vi "Focus Gray Image Stack.vi"(4 "Height Map":T1, 6 "Focused Image":T1, 8 "error in (no error)":errorcluster, 10 "Kernel Size":i32, 11 "Image Stack":T1[](array[typedef])) -> (0 "error out":errorcluster, 2 "Height Map":T1(plugin-control), 3 "Focused Image":T1(plugin-control))   [LabVIEW 2013]
uses:
  <vilib>/vision/Image Controls.llb/IMAQ Image.ctl
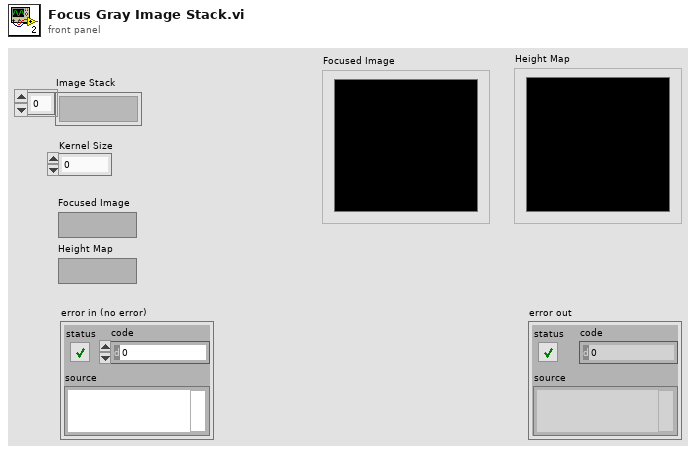
[diagram p1: front panel]
types:
  T1 = typedef "IMAQ Image.ctl" = refnum<image>
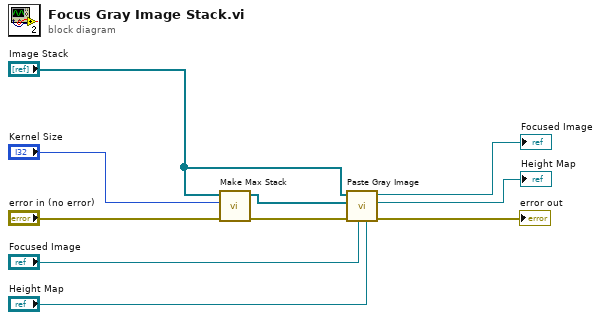
[diagram p0: block diagram]
diagram:
  n1 = call "Make Max Stack.vi"("error in (no error)"="error in (no error)", "Kernel Size"="Kernel Size", "Image Stack"="Image Stack") -> ("error out"=w10:errorcluster, "Max Stack"=w9:T1[])  [unwired: 7 in]
  n2 = call "Paste Gray Image.vi"("Height Map"="Height Map", "Focused Image"="Focused Image", "error in (no error)"=w10, "Max Image Stack"=w9, "Image Stack"="Image Stack") -> ("error out"=→"error out":errorcluster, "Height Map"=→"Height Map":T1, "Focused Image"=→"Focused Image":T1)  [unwired: 4 in]
